vi "Find Event Frame.vi"(8 "error in":errorcluster, 9 "Broadcast?":bool, 10 "VI in":refnum<vi>, 11 "Application Instance":refnum<vi>) -> (0 "error out":errorcluster)   [LabVIEW 2019, in "Panther Dashboard.lvlib"]
uses:
  Panther Dashboard.lvlib
  <vilib>/Utility/traverseref.llb/TRef TravTarget.ctl
  <vilib>/Utility/traverseref.llb/VI Scripting - Traverse.lvlib
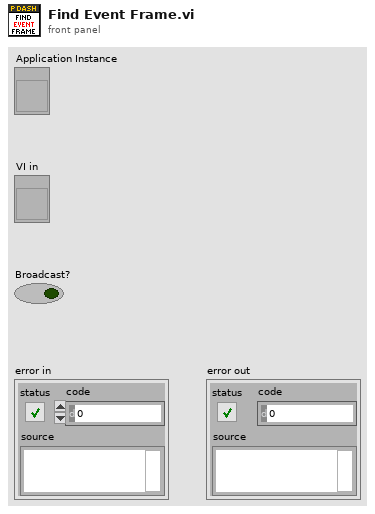
[diagram p1: front panel]
types:
  T1 = typedef "TRef TravTarget.ctl" = enum16{"FP", "BD", "Other"}
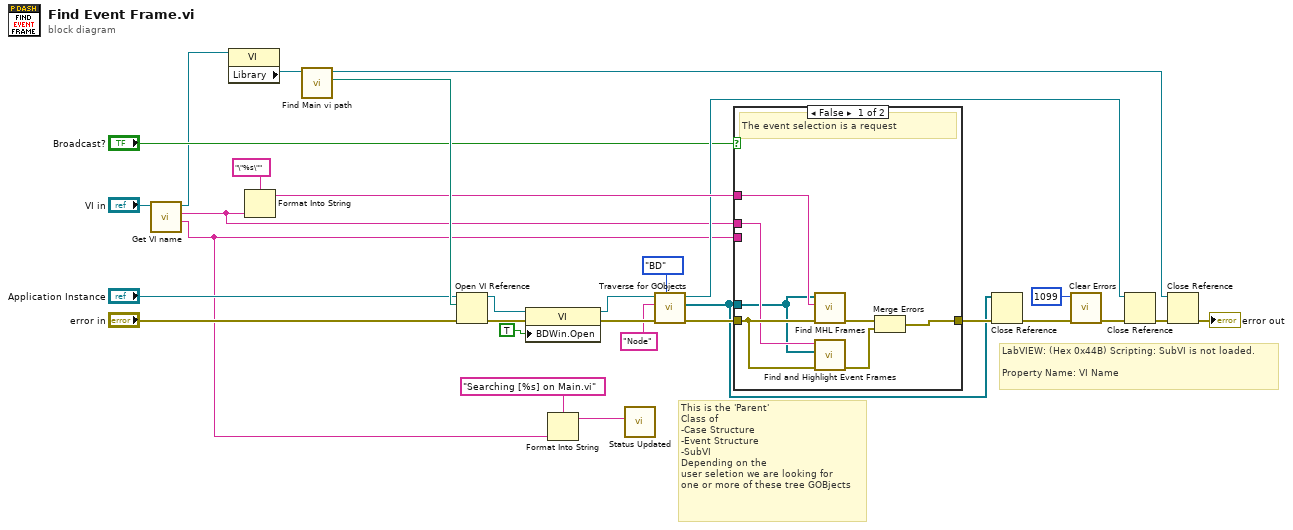
[diagram p0: block diagram]
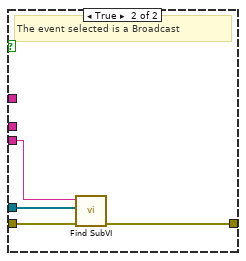
[diagram p2: hidden frame]
diagram:
  # "This is the 'Parent'\nClass of \n-Case Structure\n-Event Structure\n-SubVI\nDepending on the\nuser seletion we are looking for\none or more of these tree GOBjects"
  # "LabVIEW: (Hex 0x44B) Scripting: SubVI is not loaded.\n\nProperty Name: VI Name"
  n1 = call "Get VI name.vi"("VI in"="VI in") -> ("Full Vi Name"=w5:string, "Plain Name"=w9:string, "VI out"=w7:refnum<vi>)  [unwired: 8 in]
  n2 = property class="VI"(reference=w7) -> ("Library"=w8:refnum<vi>)  [unwired: 1 in, 2 out]
  n3 = Format Into String(format string="\"%s\"", w9) -> (resulting string=w17:string)  [unwired: 2 in, 1 out]
  n4 = call "Find Main vi path.vi"("Library in"=w8) -> ("Main vi Path"=w21:path, "Library out"=w19:refnum<vi>)  [unwired: 9 in]
  n5 = Open VI Reference(application reference (local)="Application Instance", vi path=w21, error in (no error)="error in") -> (vi reference=w20:refnum<vi>, error out=w30:errorcluster)  [unwired: 3 in]
  n6 = property class="VI"(reference=w20, error in=w30, "BDWin.Open"=TRUE ("Block Diagram Window:Open")) -> (reference out=w13:refnum<vi>, error out=w29:errorcluster)
  n7 = Format Into String(format string="Searching [%s] on Main.vi", w5) -> (resulting string=w6:string)  [unwired: 2 in, 1 out]
  n8 = call "Status Updated.vi"("Status"=w6) -> ()  [unwired: 10 in, 1 out]
  n9 = call <vilib>:"Traverse for GObjects.vi"("Traverse Target"=TRef_TravTarget."BD", "error in (no error)"=w29, "Class Name"="Node", "VI Refnum"=w13) -> ("error out"=w28:errorcluster, "References"=w1:refnum<vi>[], "dup VI Refnum"=w12:refnum<vi>)  [unwired: 4 in, 1 out]
  n10 = case shown="False" "Broadcast?" {
    tunnel: w17 -> [w33 _]
    tunnel: w28 -> [w37 w41]
    tunnel: w1 -> [w31 w38]
    tunnel: w5 -> [_ w39]
    tunnel: w9 -> [w32 _]
    tunnel: [w35 w40] -> w24
    frame False {
      # "The event selection is a request"
      n11 = call "Find MHL Frames.vi"("error in"=w37, "Event Name"=w33, "References"=w31) -> ("error out"=w36:errorcluster)  [unwired: 8 in]
      n12 = call "Find and Highlight Event Frames.vi"("error in"=w37, "References"=w31, "Event Name"=w32) -> ("error out"=w34:errorcluster)  [unwired: 8 in]
      n13 = Merge Errors(w36, w34) -> (w35:errorcluster)
    }
    frame True {
      # "The event selected is a Broadcast"
      n14 = call "Find SubVI.vi"("error in"=w41, "References"=w38, "Full Vi Name"=w39) -> ("error out"=w40:errorcluster)  [unwired: 8 in]
    }
  }
  n15 = Close Reference(reference=w1, error in (no error)=w24) -> (error out=w2:errorcluster)
  n16 = call <vilib>:"Clear Errors.vi"("error in (no error)"=w2, "specific error code to clear (0: all)"=1099) -> ("error out"=w23:errorcluster)  [unwired: 4 in, 1 out]
  n17 = Close Reference(reference=w12, error in (no error)=w23) -> (error out=w26:errorcluster)
  n18 = Close Reference(reference=w19, error in (no error)=w26) -> (error out=→"error out":errorcluster)
